vi "Send Request to Module.vi"(4 "Priority Message? (F)":bool, 8 "error in (no error)":errorcluster, 10 "Request":variant, 11 "Controller in":refnum<class "Controller.lvclass">) -> (0 "error out":errorcluster, 2 "Request (duplicate)":variant, 3 "Controller out":refnum<class "Controller.lvclass">)   [LabVIEW 2020, in "Controller.lvlib" / "Controller.lvclass"]
uses:
  Controller.lvclass
  Controller.lvclass/Controller.ctl
  RPC/TypeDefs/Request.ctl
  <vilib>/Utility/error.llb/Error Cluster From Error Code.vi
  <vilib>/ErrorRing/Error Ring.xnode
  RPC.lvlib
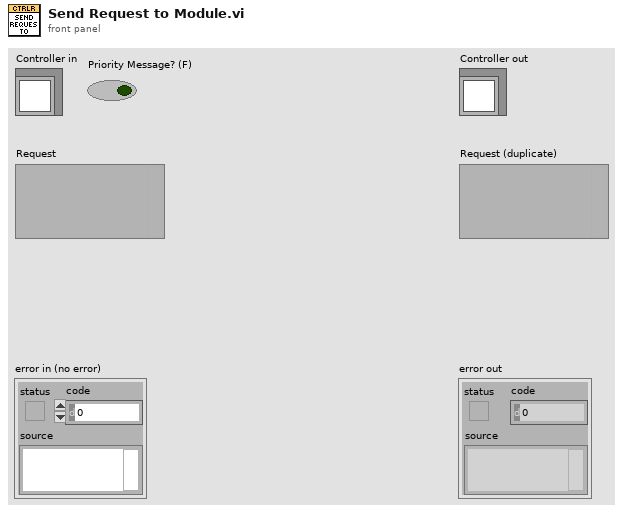
[diagram p1: front panel]
types:
  T1 = typedef "RPC.lvlib/Request.ctl" = cluster{"Method":string, "Params":variant}
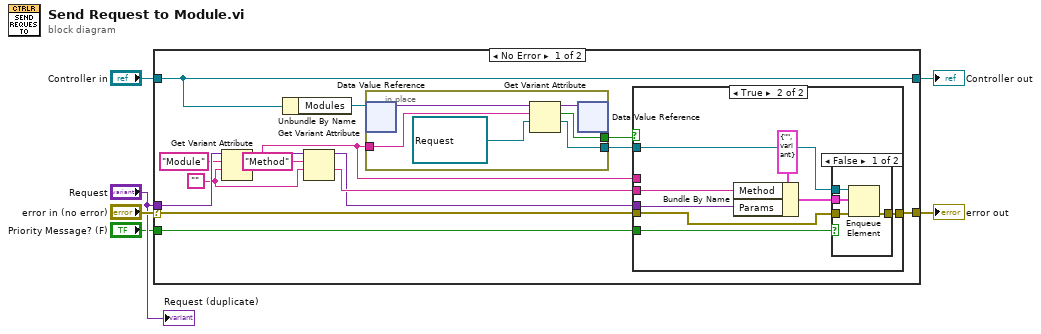
[diagram p0: block diagram]
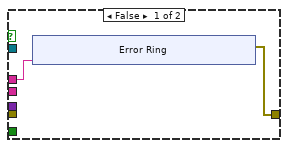
[diagram p2: hidden frame]
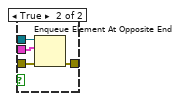
[diagram p3: hidden frame]
diagram:
  n1 = case shown="No Error" "error in (no error)" {
    selector: "error in (no error)" -> [w20 w54]
    tunnel: [w19 w54] -> w5
    tunnel: [w21 w53] -> w3
    tunnel: "Controller in" -> [w21 w53]
    tunnel: "Request" -> [w14 _]
    tunnel: "Priority Message? (F)" -> [w18 _]
    frame No Error {
      w9 = ""
      n2 = Get Variant Attribute(Variant=w14, name="Module", default value (empty Variant)=w9) -> (duplicate Variant=w11:variant, value=w12:string)  [unwired: 1 in, 2 out]
      n3 = Unbundle By Name(w21) -> ("Modules"=w17:refnum<data-value>)
      n4 = Get Variant Attribute(Variant=w11, name="Method", default value (empty Variant)=w9) -> (duplicate Variant=w7:variant, value=w8:string)  [unwired: 1 in, 2 out]
      n5 = in-place {
        in-place-border: w12 -> [w51]
        in-place-border: [w50] -> w16
        in-place-border: [w49] -> w15
        n6 = in-place-dvr #1(w17) -> (w52:variant)  [unwired: 1 out]
        n7 = Get Variant Attribute(Variant=w52, name=w51, default value (empty Variant)=refnum<queue> refnum ("queue out")) -> (duplicate Variant=w48:variant, found=w49:bool, value=w50:refnum<queue>)  [unwired: 1 in, 1 out]
        n8 = in-place-dvr #1(w48) -> ()  [unwired: 2 out]
      }
      n9 = case shown="True" w15 {
        tunnel: w20 -> [_ w38]
        tunnel: [w23 w37] -> w19
        tunnel: w8 -> [_ w34]
        tunnel: w7 -> [_ w33]
        tunnel: w18 -> [_ w31]
        tunnel: w16 -> [_ w36]
        tunnel: w12 -> [w22 _]
        frame False {
          n10 = xnode "Error Ring"("parameter 0"=w22) -> ("error out"=w23:errorcluster)
        }
        frame True {
          n11 = Bundle By Name(cluster=T1 {"Method"="", "Params"=variant} ("element"), "Method"=w34, "Params"=w33) -> (w32:T1)
          n12 = case shown="False" w31 {
            tunnel: w38 -> [w42 w46]
            tunnel: [w41 w45] -> w37
            tunnel: w36 -> [w40 w44]
            tunnel: w32 -> [w39 w43]
            frame False {
              n13 = Enqueue Element(queue=w40, element=w39, error in (no error)=w42) -> (error out=w41:errorcluster)  [unwired: 1 in, 2 out]
            }
            frame True {
              n14 = Enqueue Element At Opposite End(queue=w44, element=w43, error in (no error)=w46) -> (error out=w45:errorcluster)  [unwired: 1 in, 2 out]
            }
          }
        }
      }
    }
    frame Error {
    }
  }
  "error out" <- w5
  "Controller out" <- w3
  "Request (duplicate)" <- "Request"
